vi "Read roomNumber.vi"(8 "error in (no error)":errorcluster, 11 "Room in":refnum<class "Room.lvclass">) -> (0 "error out":errorcluster, 2 "roomNumber":i32, 3 "Room out":refnum<class "Room.lvclass">)   [LabVIEW 2016, in "Room.lvclass"]
uses:
  Room.lvclass
  Room.lvclass/Room.ctl
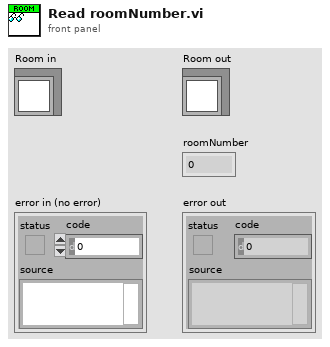
[diagram p1: front panel]
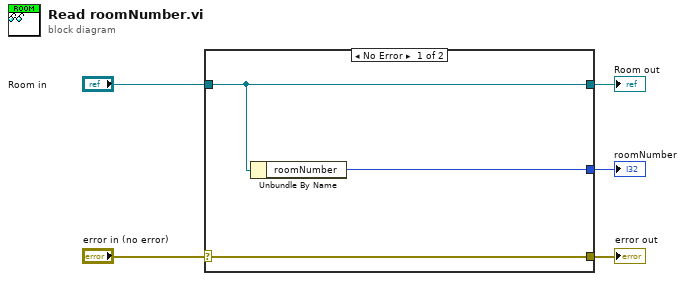
[diagram p0: block diagram]
diagram:
  n1 = case shown="No Error" "error in (no error)" {
    selector: "error in (no error)" -> [w8 w9]
    tunnel: [w8 w9] -> w4
    tunnel: [w7 w10] -> w2
    tunnel: "Room in" -> [w7 w10]
    tunnel: [w6 _] -> w1
    frame No Error {
      n2 = Unbundle By Name(w7) -> ("roomNumber"=w6:i32)
    }
    frame Error {
    }
  }
  "error out" <- w4
  "Room out" <- w2
  "roomNumber" <- w1
